vi "Generate Timestamped Filepath.vi"() -> ()   [LabVIEW 2020]
panel:
  out "timestamped relative filepath":path
  in  "appended filename":string
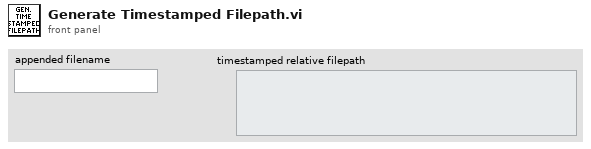
[diagram p1: front panel]
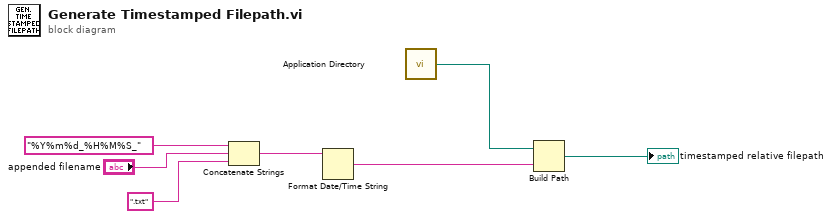
[diagram p0: block diagram]
diagram:
  n1 = Concatenate Strings "Concatenate Strings"("%Y%m%d_%H%M%S_" ("string"), "appended filename", ".txt" ("string")) -> (w4:string)
  n2 = Format Date/Time String(time format string (%c)=w4) -> (date/time string=w3:string)  [unwired: 2 in]
  n3 = call <vilib>:"Application Directory.vi"() -> ("Application Directory"=w2:path)
  n4 = Build Path(base path=w2, name or relative path=w3) -> (appended path=→"timestamped relative filepath":path)
